vi "SaveConfiguration.vi"(4 "error in (no error)":errorcluster, 7 "axis in":cluster{"keyHandle":u32, "nodeId":u16}={"keyHandle"=0, "nodeId"=1}) -> (0 "error out":errorcluster, 3 "axis out":cluster{"keyHandle":u32, "nodeId":u16}={"keyHandle"=0, "nodeId"=1})   [LabVIEW 2018]
doc: "<B>SaveConfiguration</B> saves changed parameter settings and reset the device."
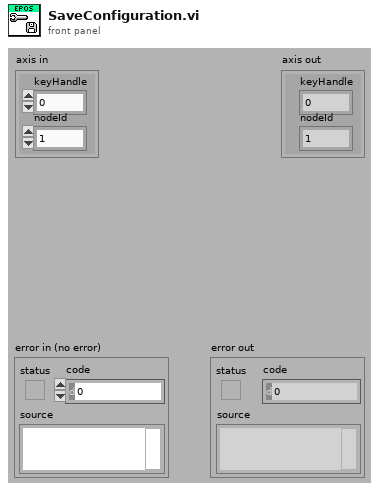
[diagram p1: front panel]
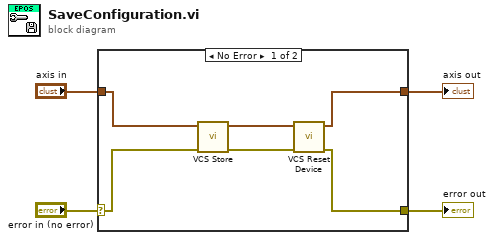
[diagram p0: block diagram]
diagram:
  n1 = case shown="No Error" "error in (no error)" {
    selector: "error in (no error)" -> [w7 w12]
    tunnel: [w5 w12] -> w3
    tunnel: [w8 w11] -> w2
    tunnel: "axis in" -> [w10 w11]
    frame No Error {
      n2 = call "VCS Store.vi"("error in (no error)"=w7, "axis in"=w10) -> ("error out"=w6:errorcluster, "axis out"=w9:cluster{"keyHandle":u32, "nodeId":u16})  [unwired: 8 in]
      n3 = call "VCS Reset Device.vi"("error in (no error)"=w6, "axis in"=w9) -> ("error out"=w5:errorcluster, "axis out"=w8:cluster{"keyHandle":u32, "nodeId":u16})  [unwired: 8 in]
    }
    frame Error {
    }
  }
  "error out" <- w3
  "axis out" <- w2
